vi "Append.vi"(8 "error in (no error)":errorcluster, 10 "ClusterTree to Append":refnum<class "TreeLUT.lvclass">, 11 "ClusterTree In":refnum<class "TreeLUT.lvclass">) -> (0 "error out":errorcluster, 3 "ClusterTree out":refnum<class "TreeLUT.lvclass">)   [LabVIEW 2017, in "TreeLUT.lvclass"]
uses:
  TreeLUT.lvclass
  TreeLUT.lvclass/TreeLUT.ctl
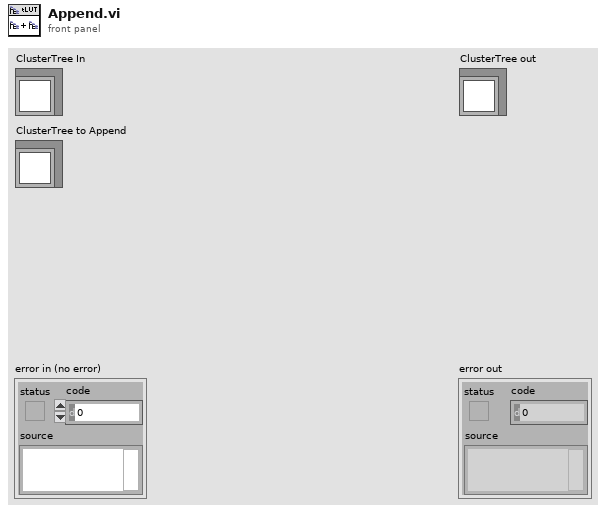
[diagram p1: front panel]
types:
  T1 = typedef "TreeLUT.lvclass/ClusterTree.ctl" = cluster{"LUT":variant, "Fields[]":string[], "Col[]":string[], "Type[]":T2[], "Indent[]":i32[]}
  T2 = typedef "NI_Data Type.lvlib/Data Type.ctl" = enum8{"Invalid Type", "Void", "I8", "I16", "I32", "I64", "U8", "U16", "U32", "U64", "Single Float", "Double Float", "Extended Float", "Single Complex", "Double Complex", "Extended Complex", "Enum U8", "Enum U16", "Enum U32", "Enum U64", "Single Float With Unit", "Double Float With Unit", "Extended Float With Unit", "Single Complex with Unit", "Double Complex with Unit", "Extended Complex with Unit", "Boolean", "String", "Path", "Picture", "Tag", "Array", "Cluster", "Variant", "LV Variant", "Waveform", "Timestamp", "Digital Waveform", "Digital Data", "ExpressData", "Refnum", "External Data", "VI", "Poly VI", "LabVIEW Class Instance", "Fixed Point"}
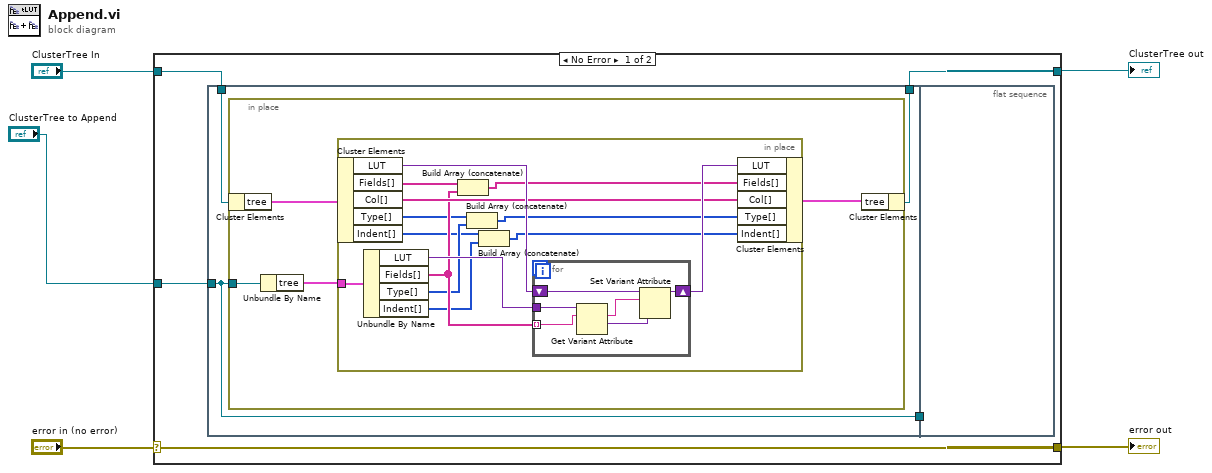
[diagram p0: block diagram]
diagram:
  n1 = case shown="No Error" "error in (no error)" {
    selector: "error in (no error)" -> [w10 w38]
    tunnel: [w10 w38] -> w4
    tunnel: [w7 w37] -> w2
    tunnel: "ClusterTree In" -> [w9 w37]
    tunnel: "ClusterTree to Append" -> [w8 _]
    frame No Error {
      n2 = flat-sequence {
        tunnel: w9 -> [w13]
        tunnel: w8 -> [w11]
        tunnel: [w12] -> w7
        tunnel: [w11] -> w6
        tunnel: w6 -> [_]
        frame #0 {
          n3 = in-place {
            in-place-border: w11 -> [w15]
            n4 = in-place-cluster #1(w13) -> ("tree"=w17:T1)
            n5 = Unbundle By Name(w15) -> ("tree"=w14:T1)
            n6 = in-place {
              in-place-border: w14 -> [w18]
              n7 = in-place-cluster #2(w17) -> ("LUT"=w31:variant, "Fields[]"=w27:string[], "Col[]"=w28:string[], "Type[]"=w24:T2[], "Indent[]"=w21:i32[])
              n8 = Unbundle By Name(w18) -> ("LUT"=w30:variant, "Fields[]"=w26:string[], "Type[]"=w22:T2[], "Indent[]"=w19:i32[])
              n9 = Build Array (concatenate)(w27, w26) -> (w25:string[])
              n10 = Build Array (concatenate)(w24, w22) -> (w23:T2[])
              n11 = Build Array (concatenate)(w21, w19) -> (w20:i32[])
              n12 = for {
                tunnel: w26 -> [w32] mode=indexing
                tunnel: w30 -> [w36]
                shift-right: [w33] -> w29
                shift-left: w31 -> [w35]
                n13 = Get Variant Attribute(Variant=w36, name=w32) -> (value=w34:variant)  [unwired: 2 in, 3 out]
                n14 = Set Variant Attribute(Variant=w35, name=w32, value=w34) -> (Variant out=w33:variant)  [unwired: 1 in, 2 out]
              }
              n15 = in-place-cluster #2("LUT"=w29, "Fields[]"=w25, "Col[]"=w28, "Type[]"=w23, "Indent[]"=w20) -> (w16:T1)
            }
            n16 = in-place-cluster #1("tree"=w16) -> (w12:refnum<class "TreeLUT.lvclass">)
          }
        }
        frame #1 {
        }
      }
    }
    frame Error {
    }
  }
  "error out" <- w4
  "ClusterTree out" <- w2
